vi "Experiment header-Generate missing stats.vi"(8 "error in (no error)":errorcluster, 11 "Experiment folder path":path) -> (0 "error out":errorcluster, 2 "STATS cluster":T1, 3 "STATS array":dbl[](array[numeric]))   [LabVIEW 2017]
uses:
  Typedefs/Test header stats cluster.ctl
  Typedefs/Logging queue element.ctl
  Typedefs/Imaging Protocols enum.ctl
  Typedefs/Frame Size.ctl
  Typedefs/Acquired points count.ctl
  Typedefs/Header file interface module functions enum.ctl
  Typedefs/Header file sections.ctl
  Typedefs/Header file type enum.ctl
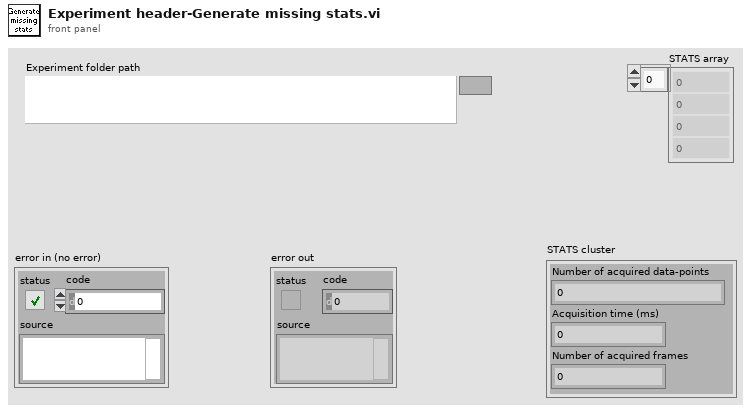
[diagram p1: front panel]
types:
  T1 = typedef "Test header stats cluster.ctl" = cluster{"Number of acquired data-points":dbl, "Acquisition time (ms)":dbl, "Number of acquired frames":dbl}
  T2 = typedef "Header file sections.ctl" = enum16{"ALL SECTIONS", "LOGIN", "GLOBAL PARAMETERS", "IMAGING MODES", "TIME SERIES", "MOTOR Z-STACK", "AOL Z-STACK", "FUNCTIONAL IMAGING", "MOVEMENT CORRECTION", "CALIBRATION", "STATISTICS", "BIOLOGY INFORMATION"}
  T3 = typedef "Header file interface module functions enum.ctl" = enum16{"Load experiment header file", "Save experiment header file", "Clear stored values", "Read stored values", "Update specific value in memory", "Update values in memory"}
  T4 = typedef "Imaging Protocols enum.ctl" = enum16{"AOL Z-Stack", "Motor Z Stack", "Functional Acquisition", "Single Plane Acquisition", "Volume Acquisition", "Live Imaging", "Live Plane Imaging", "Live Volume Imaging"}
  T5 = typedef "Logging queue element.ctl" = cluster{"Imaging Protocol":T4, "Number of Trials":u16, "Frame Size":T6, "# Averaged frames":u16, "Dwell time (us)":dbl, "Index of Z-plane":i32, "Timelapse?":bool, "Logging process is active":bool, "Speed logging enabled":bool, "tdms file ref":refnum<k34>, "path":path, "Trial Number":i32, "Expected # points acquired":bool, "Manually stopped":bool, "Ch0 data":u32[], "Ch1 data":u32[], "Ref Data":u32[], "Last trial":bool, "Ref Dwell time (us)":dbl, "# Ref Averaged frames":u16, "Ref X Length":u16, "Ref Y Length":u16, "Points acquired":T7}
  T6 = typedef "Frame Size.ctl" = u16
  T7 = typedef "Acquired points count.ctl" = cluster{"Ch0 last trial":u64, "Ch1 last trial":u64, "All trials":u64}
  T8 = typedef "Header file type enum.ctl" = enum16{"All parameters", "Params for funct acq w ROI or mscn", "Params for funct acq w rectangles", "Live imaging header parameters", "AOL Parameters"}
  T9 = typedef "Header parameters cluster-ALL.ctl" = cluster{"LOGIN":T10, "GLOBAL PARAMETERS":T11, "IMAGING MODES":T13, "TIME SERIES":T14, "MOTOR Z-STACK ":T16, "AOL Z-STACK":T17, "FUNCTIONAL IMAGING":T18, "MOVEMENT CORRECTION":T22, "CALIBRATION":T24, "STATISTICS":T25, "BIOLOGY INFORMATION":T26}
  T10 = typedef "Header params -Login.ctl" = cluster{"User":string, "Profile":string, "Software Version":string, "Experiment Date Time":timestamp}
  T11 = typedef "Header params-Global Parameters.ctl" = cluster{"MicroscopeID":string, "Microscope Type":string, "Objective":string, "Field of View (um)":dbl, "Fill time (us)":dbl, "Experiment Type":T12, "Stimuli Trigger":bool, "Speed Logging":bool}
  T12 = typedef "Experiment Type.ctl" = enum16{"In vivo", "In vitro", "Testing", "Calibration", "Other"}
  T13 = typedef "Header params-Imaging Modes.ctl" = cluster{"Time Series":bool, "Motor Zstack":bool, "AOL Zstack":bool, "Functional Imaging":bool}
  T14 = typedef "Header params-Time Series.ctl" = cluster{"Basic Image meta data":T15, "AOL z":dbl}
  T15 = typedef "Header params-Basic image meta data.ctl" = cluster{"Wavelength (nm)":dbl, "# averaged frames":dbl, "laser power (%)":dbl, "Pockels":dbl, "pixel dwell time (us)":dbl, "pmt 1":dbl, "pmt 2":dbl, "back apperture":dbl, "zoom":dbl, "field of view":dbl, "Frame Size":T6, "AOL x centre":dbl, "AOL y centre":dbl, "Stage x position":dbl, "Stage y position":dbl, "Stage z position":dbl}
  T16 = typedef "Header params-Motor Z-stack.ctl" = cluster{"Hdr Basic Image meta data":T15, "Z Start":dbl, "Z Stop":dbl, "No of Planes":i32}
  T17 = typedef "Header params-AOL Z-stack.ctl" = cluster{"Hdr Basic Image meta data":T15, "Z Start":dbl, "Z Stop":dbl, "No of Planes":i32}
  T18 = typedef "Header params-Functional Imaging.ctl" = cluster{"Functional Mode":T19, "Pockels Modulation":bool, "Number of pois":dbl, "Number of miniscans":dbl, "Number of cycles":dbl, "Number of trials":dbl, "Miniscan dwell time per pixel (us)":dbl, "Number of pixels in miniscan":dbl, "poi dwell time":dbl, "Rectangle ROI length":dbl, "Rectangle ROI height":dbl, "AOL Mode":T20, "Plane Mode":T21, "video length (sec)":dbl, "Frame rate (fps)":dbl, "Stimuli Timing (usec)":dbl, "Acquisition Length":dbl, "Basic Image meta data":T15, "Z Start (um)":dbl, "Z Stop (um)":dbl}
  T19 = typedef "Functional Mode.ctl" = enum16{"Point", "Line", "Patch", "Plane", "Volume"}
  T20 = typedef "AOL modes.ctl" = enum16{"Raster", "Structural", "Pointing", "Mini Scan", "Alignment"}
  T21 = typedef "Plane Mode.ctl" = u16
  T22 = typedef "Header params-Movement correction.ctl" = cluster{"Movement Correction":bool, "Axial Reference":bool, "Reference X Pixels":dbl, "Reference Y Pixels":dbl, "Reference Source":T23, "Reference dwell time (us)":dbl, "Number of Z lines":dbl, "Size of Z pixels":dbl, "Axial Pixels":dbl, "Reference Zoom":dbl, "Reference Average":dbl, "Proportional Scale":dbl, "Integral Scale":dbl, "Proportional Scale Z":dbl, "Integral Scale Z":dbl, "Scan Interval":dbl, "Ref Plot Refresh Rate":dbl}
  T23 = typedef "Reference source.ctl" = enum16{"Green channel", "Red channel"}
  T24 = typedef "Header params-Calibration Setup.ctl" = cluster{"Pockels Calibration File":path, "Calibration_ini file":path, "Setup_ini file":path}
  T25 = typedef "Header params-statistics.ctl" = cluster{"Z-stack duration (sec)":dbl, "Number of acquired data-points":dbl, "Acquisition time (ms)":dbl, "Number of acquired frames":dbl}
  T26 = typedef "Biology Information.ctl" = cluster{"Animal Code or Name":string, "Animal DoB":string, "Animal Age":string, "Animal Sex":string, "Animal Weight":string, "Date of Injection":string, "Date of Implant":string, "Site of Injection":string, "Animal Ear Notch":string, "AAV constructs":string, "Genetic background":string, "Optical reporter":string, "Region of brain imaged":string, "Other \ncomments":string}
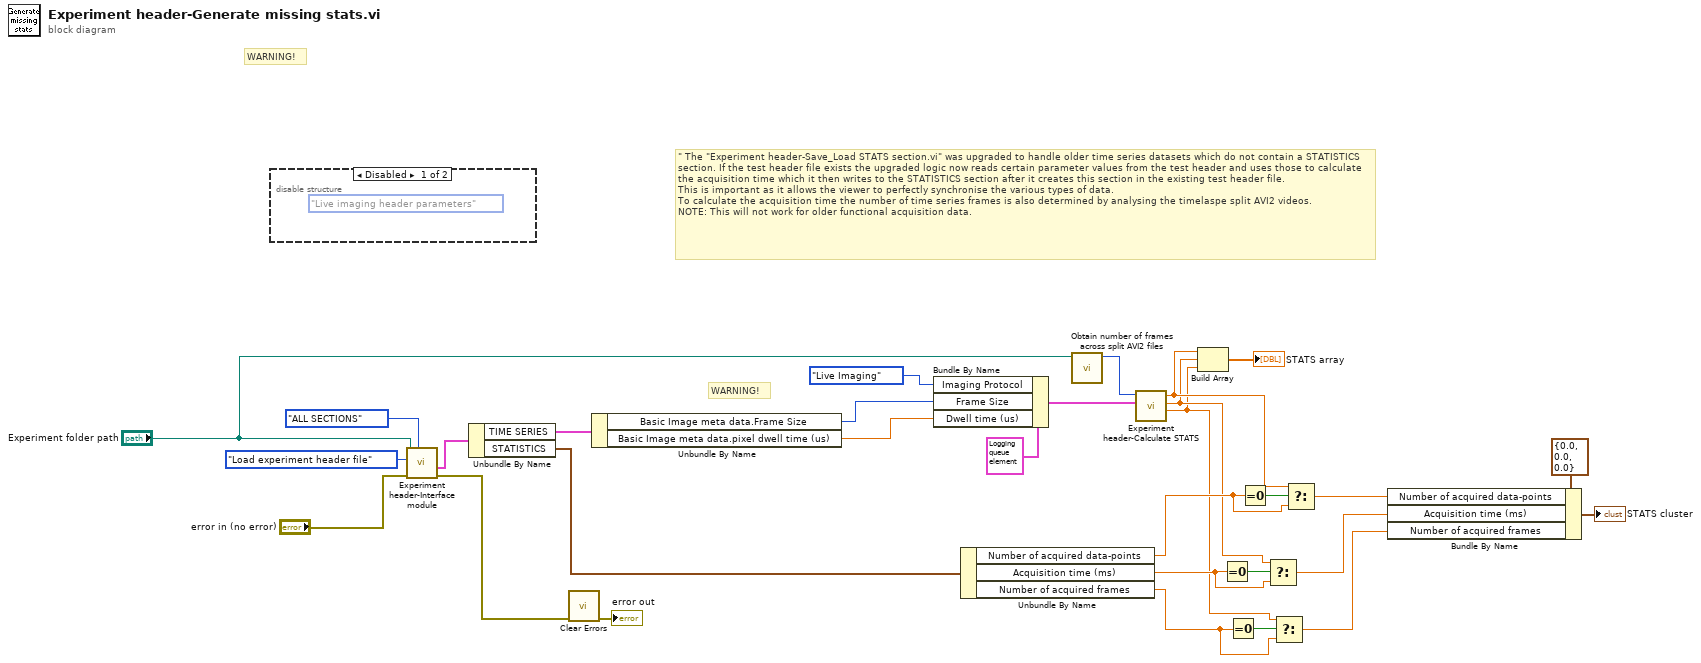
[diagram p0: block diagram]
diagram:
  # "WARNING!"
  # "WARNING!"
  # "\"\tThe \"Experiment header-Save_Load STATS section.vi\" was upgraded to handle older time series datasets which do not contain a STATISTICS section. If the test header file exists the upgraded logic now reads certain parameter values from the test header and uses those to calculate the acquisition time which it then writes to the STATISTICS section after it creates this section in the existing test header file. \nThis is important as it allows the viewer to perfectly synchronise the various types of data.\nTo calculate the acquisition time the number of time series frames is also determined by analysing the timelaspe split AVI2 videos. \nNOTE: This will not work for older functional acquisition data."
  n1 = disable-structure shown="Disabled" {
    frame Disabled {
      (unwired) Header_file_type_enum."Live imaging header parameters" ("Header file type")
    }
    frame Enabled {
    }
  }
  n2 = call "Experiment header-Interface module.vi"("Header file sections"=Header_file_sections."ALL SECTIONS", "error in (no error)"="error in (no error)", "Function"=Header_file_interface_module_functions_enum."Load experiment header file", "Experiment data folder path"="Experiment folder path") -> ("error out"=w21:errorcluster, "All header parameters out"=w23:T9)  [unwired: 6 in]
  n3 = Unbundle By Name(w23) -> ("TIME SERIES"=w22:T14, "STATISTICS"=w15:T25)
  n4 = call <vilib>:"Clear Errors.vi"("error in (no error)"=w21) -> ("error out"=→"error out":errorcluster)  [unwired: 5 in, 1 out]
  n5 = Unbundle By Name(w22) -> ("Basic Image meta data.Frame Size"=w19:T6, "Basic Image meta data.pixel dwell time (us)"=w20:dbl)
  n6 = Bundle By Name(cluster=T5 {"Imaging Protocol"=enum."Live Imaging", "Number of Trials"=0, "Frame Size"=0, "# Averaged frames"=0, "Dwell time (us)"=0.1, "Index of Z-plane"=0, "Timelapse?"=FALSE, "Logging process is active"=FALSE, "Speed logging enabled"=FALSE, "tdms file ref"=refnum, "path"=path "", "Trial Number"=0, "Expected # points acquired"=FALSE, "Manually stopped"=FALSE, "Ch0 data"=[], "Ch1 data"=[], "Ref Data"=[], "Last trial"=FALSE, "Ref Dwell time (us)"=0.0, "# Ref Averaged frames"=0, "Ref X Length"=0, "Ref Y Length"=0, "Points acquired"={"Ch0 last trial"=0, "Ch1 last trial"=0, "All trials"=0}} ("Logging queue element"), "Imaging Protocol"=Imaging_Protocols_enum."Live Imaging", "Frame Size"=w19, "Dwell time (us)"=w20) -> (w30:T5)
  n7 = Unbundle By Name(w15) -> ("Number of acquired data-points"=w13:dbl, "Acquisition time (ms)"=w10:dbl, "Number of acquired frames"=w7:dbl)
  n8 = call "Obtain number of frames across split AVI2 files.vi"("Experiment folder path"="Experiment folder path") -> ("Number of Frames (across all split videos of a single channel)"=w27:u32)  [unwired: 9 in, 1 out]
  n9 = call "Experiment header-Calculate STATS.vi"("Logging queue element"=w30, "Timelapse frames saved"=w27) -> ("Number of acquired frames"=w2:dbl, "Acquisition time (ms)"=w3:dbl, "Total number of points acquired (Ch0)"=w4:dbl)  [unwired: 7 in]
  n10 = Build Array(w4, w3, w2) -> (→"STATS array":dbl[])
  n11 = Equal To 0?(x=w10) -> (x = 0?=w11:bool)
  n12 = Equal To 0?(x=w7) -> (x = 0?=w8:bool)
  n13 = Equal To 0?(x=w13) -> (x = 0?=w14:bool)
  n14 = Select(t=w3, s=w11, f=w10) -> (s? t:f=w9:dbl)
  n15 = Select(t=w2, s=w8, f=w7) -> (s? t:f=w6:dbl)
  n16 = Select(t=w4, s=w14, f=w13) -> (s? t:f=w12:dbl)
  n17 = Bundle By Name(cluster=T1 {"Number of acquired data-points"=0.0, "Acquisition time (ms)"=0.0, "Number of acquired frames"=0.0} ("Read values 2"), "Number of acquired data-points"=w12, "Acquisition time (ms)"=w9, "Number of acquired frames"=w6) -> (→"STATS cluster":T1)
